vi "Actor Core.vi"(8 "error in":errorcluster, 11 "My Application":refnum<class "CoordinatorUI.lvclass">) -> (0 "error out":errorcluster, 3 "Actor out":refnum<class "Actor.lvclass">)   [LabVIEW 2014, in "CoordinatorUI.lvlib" / "CoordinatorUI.lvclass"]
doc: "This is Actor Core.vi, the main message handling loop for Actors. An actor usually just sits in this loop and processes messages as they arrive. Any error returned by the message Do.vi call will stop the loop, with error code 43 as the canonical signal to stop with no error sent to caller. Descendants may override that in Handle Error.vi."
uses:
  CoordinatorUI.lvclass
  <vilib>/ActorFramework/Actor/Actor.lvclass
  <vilib>/ActorFramework/Stop Msg/Stop Msg.lvclass
  labview/1512/State Pattern Actor Example/Process States/Process State Messages/Go to Running Msg/Go to Running Msg.lvclass
  labview/1512/State Pattern Actor Example/Process States/Process State Messages/Go to Idle Msg/Go to Idle Msg.lvclass
  labview/1512/State Pattern Actor Example/Process States/Process State Messages/Request Update from Process Msg/Request Update from Process Msg.lvclass
  Wrapper_lib/zsActor/ActorWrapper.lvclass
  States_lib/Idle/Ready.lvclass
panel:
  in  "Message to State 3":bool
  in  "Message to State 2":bool
  in  "stop signal":bool
  out "Event Log":string
  in  "DNL_Stop":bool
  in  "Message to State":bool
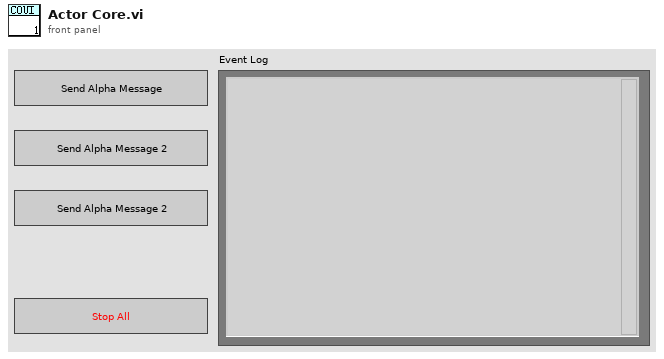
[diagram p1: front panel]
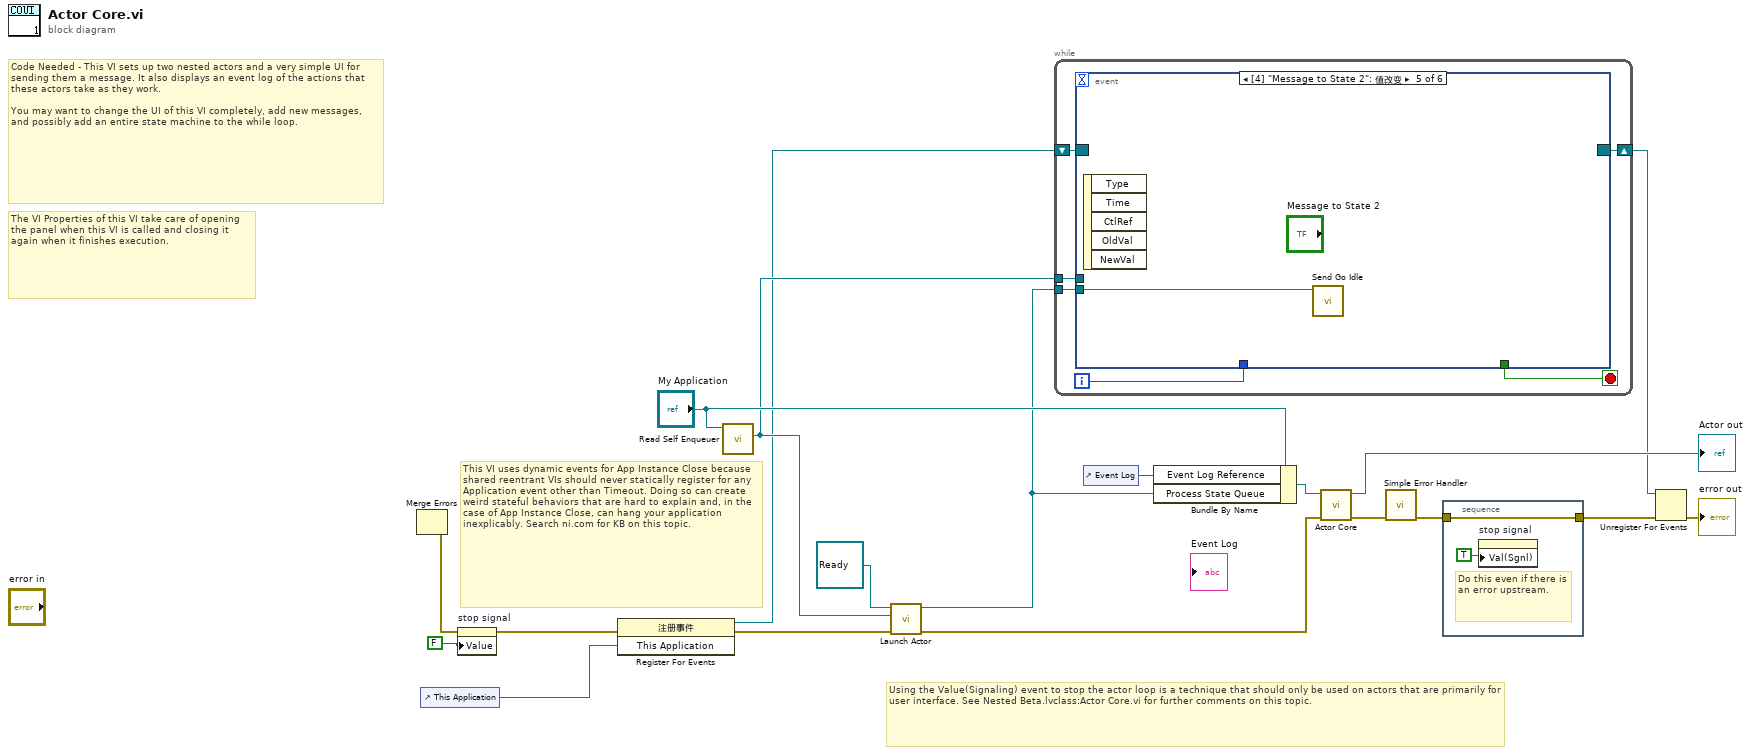
[diagram p0: block diagram]
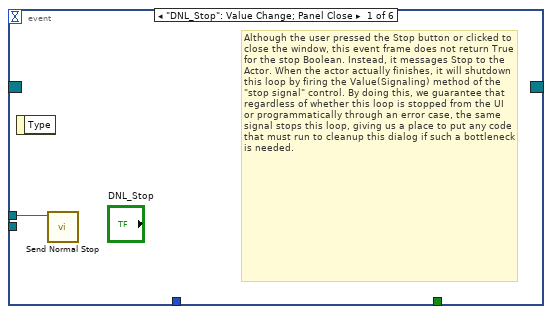
[diagram p2: hidden frame]
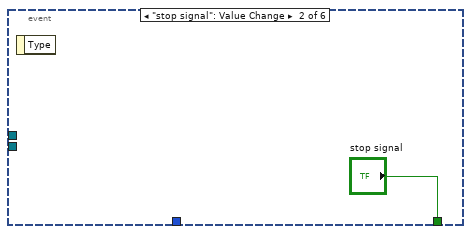
[diagram p3: hidden frame]
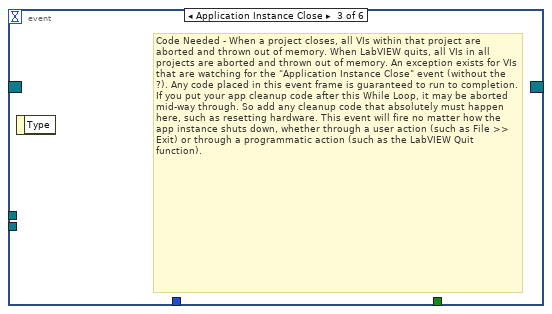
[diagram p4: hidden frame]
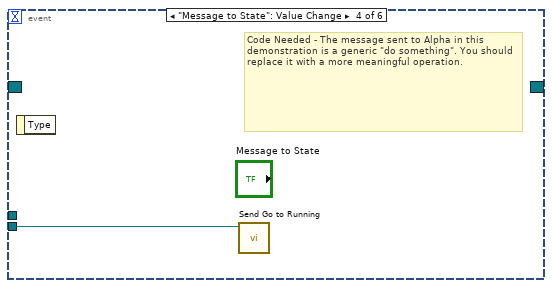
[diagram p5: hidden frame]
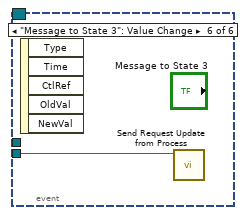
[diagram p6: hidden frame]
diagram:
  # "This VI uses dynamic events for App Instance Close because shared reentrant VIs should never statically register for any Application event other than Timeout. Doing so can create weird stateful behaviors that are hard to explain and, in the case of App Instance Close, can hang your application inexplicably. Search ni.com for KB on this topic."
  # "The VI Properties of this VI take care of opening the panel when this VI is called and closing it again when it finishes execution."
  # "Using the Value(Signaling) event to stop the actor loop is a technique that should only be used on actors that are primarily for user interface. See Nested Beta.lvclass:Actor Core.vi for further comments on this topic."
  # "Code Needed - This VI sets up two nested actors and a very simple UI for sending them a message. It also displays an event log of the actions that these actors take as they work. \n\nYou may want to change the UI of this VI completely, add new messages, and possibly add an entire state machine to the while loop."
  n1 = Merge Errors() -> (w12:errorcluster)  [unwired: 3 in]
  n2 = control-ref of="This Application"() -> (w3:refnum<vi>)
  n3 = property on="stop signal" class="Bool (严格)"(error in=w12, "Value"=FALSE ("stop")) -> (error out=w5:errorcluster)  [unwired: 1 in, 1 out]
  n4 = register-events(error in=w5, w3) -> (reference out=w9:refnum<event-registration>, error out=w4:errorcluster)  [unwired: 1 in]
  n5 = call <vilib>:"Read Self Enqueuer.vi"("Actor"="My Application") -> ("Self Enqueuer"=w14:refnum<class "Message Enqueuer.lvclass">)  [unwired: 10 in]
  n6 = call <vilib>:"Launch Actor.vi"("error in (no error)"=w4, "Actor-to-Caller Enqueuer"=w14, "Actor"=refnum<class "Ready.lvclass"> refnum ("States.lvlib:Ready.lvclass")) -> ("error out"=w18:errorcluster, "Caller-To-Actor Enqueuer"=w2:refnum<class "Message Enqueuer.lvclass">)  [unwired: 7 in]
  n7 = while {
    tunnel: w14 -> [w25]
    tunnel: w2 -> [w24]
    shift-right: [w20] -> w8
    shift-left: w9 -> [w21]
    i -> [w22]
    stop <- w23 stop-if-true
    n8 = event shown="[4] \"Message to State 2\": 值改变" {
      selector: w21 -> [_ _ _ _ _ _]
      dyn-events: [_ _ _ _ _ _] -> w20
      timeout: _ -> [_ _ _ _ _ _]
      tunnel: w25 -> [w26 _ _ _ _ _]
      tunnel: w24 -> [_ _ _ w28 w29 w30]
      tunnel: [_ "stop signal" _ _ _ _] -> w23
      tunnel: w22 -> [_ _ _ _ _ _]
      event "DNL_Stop": Value Change; Panel Close {
        # "Although the user pressed the Stop button or clicked to close the window, this event frame does not return True for the stop Boolean. Instead, it messages Stop to the Actor. When the actor actually finishes, it will shutdown this loop by firing the Value(Signaling) method of the \"stop signal\" control. By doing this, we guarantee that regardless of whether this loop is stopped from the UI or programmatically through an error case, the same signal stops this loop, giving us a place to put any code that must run to cleanup this dialog if such a bottleneck is needed."
        n9 = event-data() -> ()  [unwired: 1 in, 1 out]
        n10 = call <vilib>:"Send Normal Stop.vi"("Message Enqueuer"=w26) -> ()  [unwired: 10 in, 1 out]
      }
      event "stop signal": Value Change {
        n11 = event-data() -> ()  [unwired: 1 in, 1 out]
      }
      event Application Instance Close {
        # "Code Needed - When a project closes, all VIs within that project are aborted and thrown out of memory. When LabVIEW quits, all VIs in all projects are aborted and thrown out of memory. An exception exists for VIs that are watching for the \"Application Instance Close\" event (without the ?). Any code placed in this event frame is guaranteed to run to completion. If you put your app cleanup code after this While Loop, it may be aborted mid-way through. So add any cleanup code that absolutely must happen here, such as resetting hardware. This event will fire no matter how the app instance shuts down, whether through a user action (such as File >> Exit) or through a programmatic action (such as the LabVIEW Quit function)."
        n12 = event-data() -> ()  [unwired: 1 in, 1 out]
      }
      event "Message to State": Value Change {
        # "Code Needed - The message sent to Alpha in this demonstration is a generic \"do something\". You should replace it with a more meaningful operation."
        n13 = event-data() -> ()  [unwired: 1 in, 1 out]
        n14 = call "Send Go to Running.vi"("Message Enqueuer"=w28) -> ()  [unwired: 9 in, 2 out]
      }
      event "Message to State 2": Value Change {
        n15 = event-data() -> ()  [unwired: 1 in, 5 out]
        n16 = call "Send Go Idle.vi"("Message Enqueuer"=w29) -> ()  [unwired: 9 in, 2 out]
      }
      event "Message to State 3": Value Change {
        n17 = event-data() -> ()  [unwired: 1 in, 5 out]
        n18 = call "Send Request Update from Process.vi"("Message Enqueuer"=w30) -> ()  [unwired: 9 in, 2 out]
      }
    }
  }
  n19 = control-ref of="Event Log"() -> (w15:refnum<vi>)
  n20 = Bundle By Name(cluster="My Application", "Event Log Reference"=w15, "Process State Queue"=w2) -> (w16:refnum<class "CoordinatorUI.lvclass">)
  n21 = call-parent "Actor Core.vi"("error in"=w18, "Actor in"=w16) -> ("error out"=w11:errorcluster, "Actor out"=→"Actor out":refnum<class "Actor.lvclass">)  [unwired: 8 in]
  n22 = call <vilib>:"Simple Error Handler.vi"("error in (no error)"=w11) -> ("error out"=w10:errorcluster)  [unwired: 4 in, 4 out]
  n23 = stacked-sequence {
    tunnel: [w31] -> w7
    tunnel: w10 -> [w31]
    frame #0 {
      # "Do this even if there is an error upstream."
      n24 = property on="stop signal" class="Bool (严格)"("Val(Sgnl)"=TRUE ("stop")) -> ()  [unwired: 2 in, 2 out]
    }
  }
  n25 = Unregister For Events(event registration refnum=w8, error in=w7) -> (error out=→"error out":errorcluster)
